vi "Add Error Core.vi"(8 "error in (no error)":errorcluster, 10 "String to Append":string, 11 "Error":T1) -> (0 "error out":errorcluster)   [LabVIEW 2021, in "pcap_Parse_Build_CIF.lvclass"]
uses:
  pcap_Parse_Build_CIF.lvclass
  pcap_Parse_Build_CIF.lvclass/pcap_Parse_Build_CIF.ctl
  <vilib>/CIF Foundation/CIF Utilities/Errors/Errors_CIF_U.lvlib
  Typedef/Errors.ctl
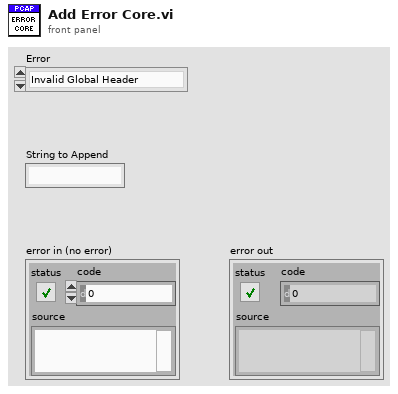
[diagram p1: front panel]
types:
  T1 = typedef "pcap_Parse_Build_CIF.lvclass/Errors.ctl" = enum16{"Invalid Global Header", "Out of Data"}
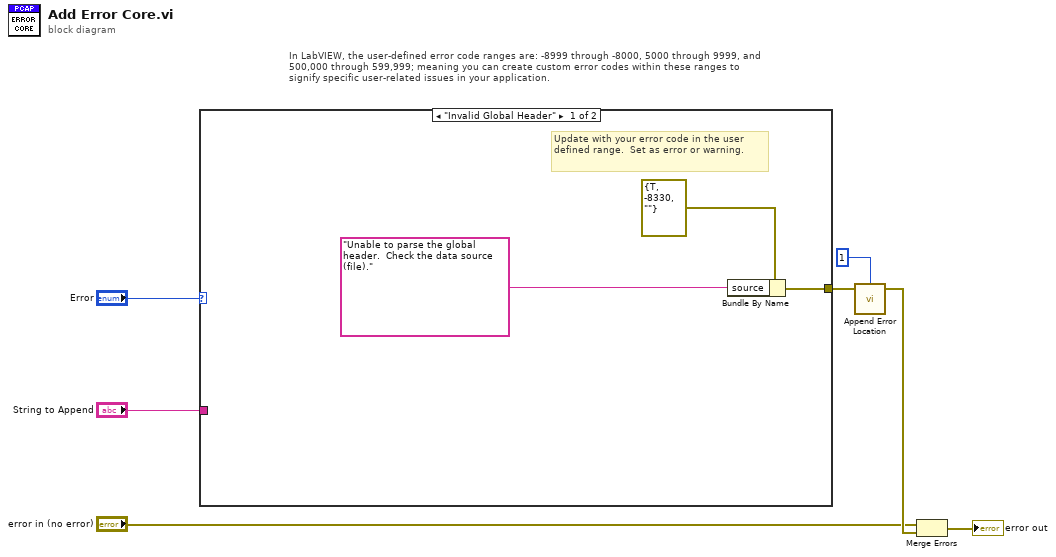
[diagram p0: block diagram]
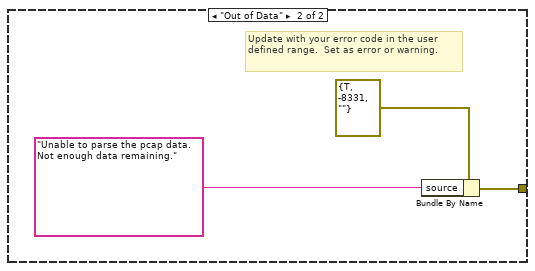
[diagram p2: hidden frame]
diagram:
  # "In LabVIEW, the user-defined error code ranges are: -8999 through -8000, 5000 through 9999, and 500,000 through 599,999; meaning you can create custom error codes within these ranges to signify specific user-related issues in your application."
  n1 = case shown="\"Invalid Global Header\"" "Error" {
    tunnel: "String to Append" -> [_ _]
    tunnel: [w9 w12] -> w6
    frame "Invalid Global Header" {
      # "Update with your error code in the user defined range.  Set as error or warning."
      n2 = Bundle By Name(cluster=errorcluster {"status"=TRUE, "code"=-8330, "source"=""} ("Invalid ID"), "source"="Unable to parse the global header.  Check the data source (file).") -> (w9:errorcluster)
    }
    frame "Out of Data" {
      # "Update with your error code in the user defined range.  Set as error or warning."
      n3 = Bundle By Name(cluster=errorcluster {"status"=TRUE, "code"=-8331, "source"=""} ("Invalid ID"), "source"="Unable to parse the pcap data.  Not enough data remaining.") -> (w12:errorcluster)
    }
  }
  n4 = call <vilib>:"Append Error Location.vi"("error in (no error)"=w6, "Chain Depth"=1) -> ("error out"=w7:errorcluster)  [unwired: 3 in]
  n5 = Merge Errors("error in (no error)", w7) -> (→"error out":errorcluster)
